vi "test_wind_rotation.vi"() -> ()   [LabVIEW 2013]
uses:
  <vilib>/Analysis/coordinate.llb/2D Cartesian Coordinate Rotation (Scalar).vi
  <vilib>/Analysis/NI_AALPro.lvlib
panel:
  out "y out":dbl
  out "x out":dbl
  in  "Dial":dbl(knob) scale format="%#1_6g"
  in  "Y pos":dbl(slide) scale=-10.0..10.0
  in  "X pos":dbl(slide) scale=-10.0..10.0
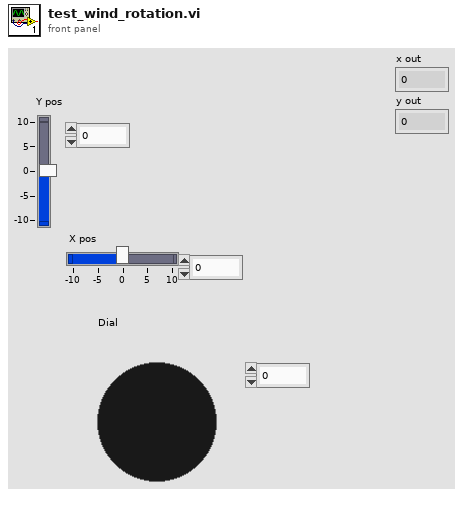
[diagram p1: front panel]
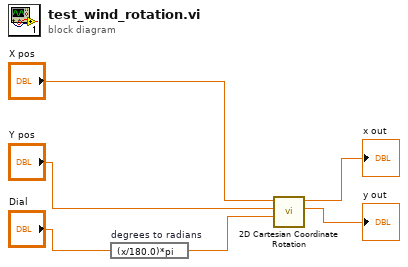
[diagram p0: block diagram]
diagram:
  n1 = expression code="(x/180.0)*pi" "degrees to radians"("Dial") -> (w3:dbl)
  n2 = call-poly <vilib>:"2D Cartesian Coordinate Rotation.vi"("theta"=w3, "y"="Y pos", "x"="X pos") -> ("y out"=→"y out":dbl, "x out"=→"x out":dbl)  [unwired: 6 in, 1 out]
